vi "ColourCheckTesting.vi"   [LabVIEW 2022 SP3]
uses:
  Reading Red.vi
  Global Red Initial.vi
  Reading Green.vi
  Global Green Initial.vi
  Reading Blue.vi
  Global Blue Initial.vi
  Global Red After Box.vi
  Global Green After Box.vi
  Global Blue After Box.vi
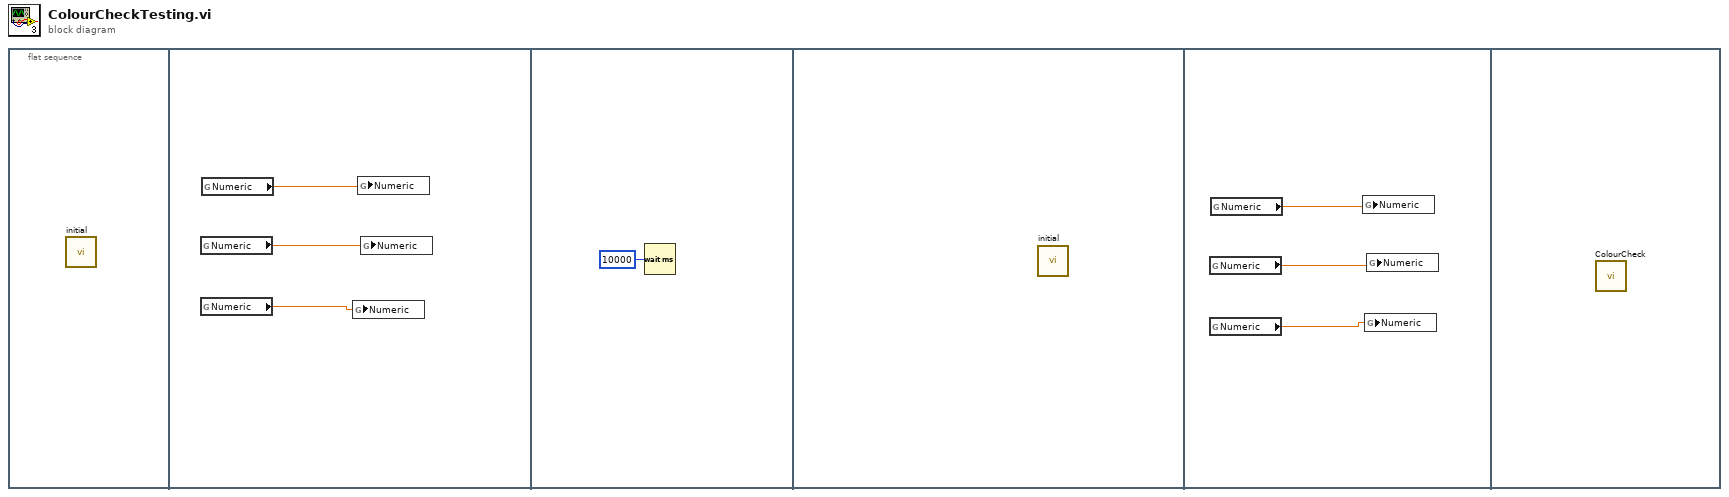
[diagram p0: block diagram]
diagram:
  n1 = flat-sequence {
    frame #0 {
      n2 = call "initial.vi"() -> ()  [unwired: 12 in]
    }
    frame #1 {
      n3 = global read "Reading Green.vi" "Numeric"() -> (w2:dbl)
      n4 = global read "Reading Blue.vi" "Numeric"() -> (w1:dbl)
      n5 = global read "Reading Red.vi" "Numeric"() -> (w3:dbl)
      n6 = global write "Global Blue Initial.vi" "Numeric"(w1) -> ()
      n7 = global write "Global Red Initial.vi" "Numeric"(w3) -> ()
      n8 = global write "Global Green Initial.vi" "Numeric"(w2) -> ()
    }
    frame #2 {
      n9 = Wait (ms)(milliseconds to wait=u32 10000) -> ()  [unwired: 1 out]
    }
    frame #3 {
      n10 = call "initial.vi"() -> ()  [unwired: 12 in]
    }
    frame #4 {
      n11 = global read "Reading Green.vi" "Numeric"() -> (w6:dbl)
      n12 = global read "Reading Blue.vi" "Numeric"() -> (w5:dbl)
      n13 = global read "Reading Red.vi" "Numeric"() -> (w7:dbl)
      n14 = global write "Global Red After Box.vi" "Numeric"(w7) -> ()
      n15 = global write "Global Blue After Box.vi" "Numeric"(w5) -> ()
      n16 = global write "Global Green After Box.vi" "Numeric"(w6) -> ()
    }
    frame #5 {
      n17 = call "ColourCheck.vi"() -> ()  [unwired: 12 in]
    }
  }
